vi "IPI_PluseTomm.vi"(10 "Radio":string, 11 "Pluse":string) -> (2 "mm":dbl, 3 "mm":string)   [LabVIEW 2015]
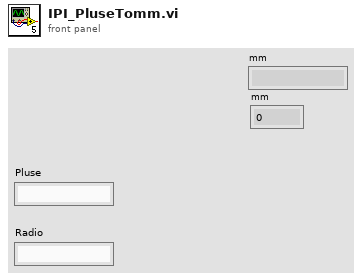
[diagram p1: front panel]
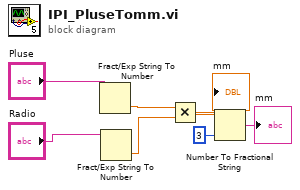
[diagram p0: block diagram]
diagram:
  n1 = Fract/Exp String To Number(string="Pluse") -> (number=w5:dbl)  [unwired: 3 in, 1 out]
  n2 = Fract/Exp String To Number(string="Radio") -> (number=w4:dbl)  [unwired: 3 in, 1 out]
  n3 = Multiply(x=w5, y=w4) -> (x*y=w3:dbl)
  "mm" <- w3
  n4 = Number To Fractional String(number=w3, precision (6)=i16 3 ("精度(6)")) -> (F-format string=→"mm":string)  [unwired: 2 in]
